vi "Verify Key Match.vi"(8 "error in (no error)":errorcluster, 10 "Shared Key":string, 11 "Attribute.Owner in":refnum<class "Attribute.Owner.lvclass">) -> (0 "error out":errorcluster, 1 "not set":bool, 2 "key matched":bool, 3 "Attribute.Owner out":refnum<class "Attribute.Owner.lvclass">)   [LabVIEW 2019, in "Attribute.Owner.lvclass"]
doc: "JKI State Machine Objects (SMO) 1.3.0.56\nJKI - JKI\nCopyright (c) 2017, JKI"
uses:
  Attribute.Owner.lvclass
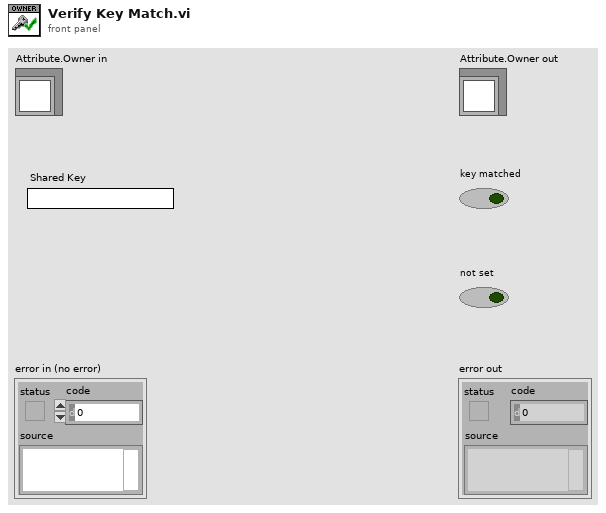
[diagram p1: front panel]
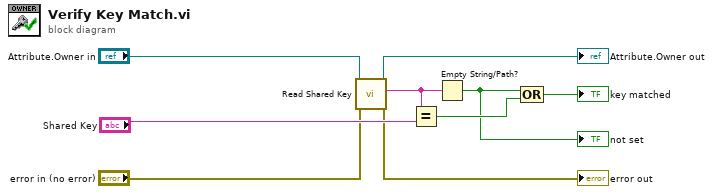
[diagram p0: block diagram]
diagram:
  n1 = call "Read Shared Key.vi"("error in (no error)"="error in (no error)", "Attribute.Owner in"="Attribute.Owner in") -> ("error out"=→"error out":errorcluster, "Shared Key"=w5:string, "Attribute.Owner out"=→"Attribute.Owner out":refnum<class "Attribute.Owner.lvclass">)  [unwired: 7 in]
  n2 = Equal?(x=w5, y="Shared Key") -> (x = y?=w4:bool)
  n3 = Empty String/Path?(string/path=w5) -> (empty?=w1:bool)
  "not set" <- w1
  n4 = Compound Arithmetic op=OR(w1, w4) -> (→"key matched":bool)
